vi "Toolbar Set Button Image (Picture).vi"(0 "Display State In":T2={"Buttons Displayed"=0, "Button States"=[], "Button Size"=0, "Button Style"=enum."Classic", "Active Button"=0, "Force Regen?"=FALSE, "Tip String Ref"=refnum}, 1 "Button Index":i32, 5 "State":T1, 7 "Picture":picture, 9 "Container State":T4, 11 "error in (no error)":errorcluster) -> (4 "Display State Out":T2={"Buttons Displayed"=0, "Button States"=[], "Button Size"=0, "Button Style"=enum."Classic", "Active Button"=0, "Force Regen?"=FALSE, "Tip String Ref"=refnum}, 15 "error out":errorcluster)   [LabVIEW 2012, in "Toolbar.xctl"]
doc: "Sets the image of specific button and state from a picture control."
uses:
  Toolbar.xctl
  <vilib>/_xctls/Container State.ctl
  Toolbar State.ctl
  Button_Class/Button.lvclass
  Button_Class/Type Defs/Button Style.ctl
  Button_Class/Type Defs/Button Status.ctl
  <vilib>/_xctls/XControlSupport.lvlib
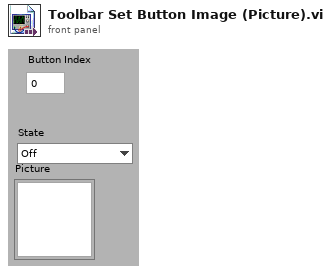
[diagram p1: front panel]
types:
  T1 = typedef "Button.lvclass/Button Status.ctl" = enum16{"Off", "Hover", "On", "Disabled"}
  T2 = typedef "Toolbar.xctl/Toolbar State.ctl" = cluster{"Buttons Displayed":i32, "Button States":refnum<class "Button.lvclass">[], "Button Size":i32, "Button Style":T3, "Active Button":i32, "Force Regen?":bool, "Tip String Ref":refnum<vi>}
  T3 = typedef "Button.lvclass/Button Style.ctl" = enum16{"System", "Modern", "Classic", "Rounded", "Silver", "Ni Theme", "Metallic"}
  T4 = typedef "XControlSupport.lvlib/Container State.ctl" = cluster{"Indicator?":bool, "Run Mode?":bool, " Refnum":refnum<vi>}
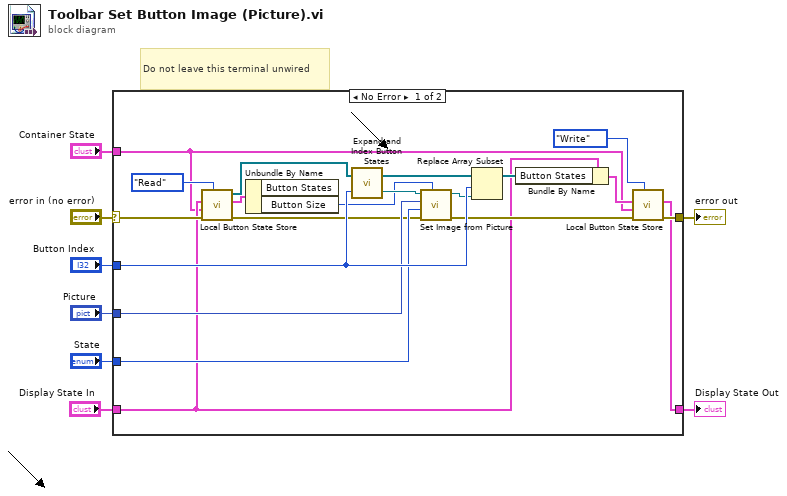
[diagram p0: block diagram]
diagram:
  # "Do not leave this terminal unwired"
  n1 = case shown="No Error" "error in (no error)" {
    selector: "error in (no error)" -> [w17 w29]
    tunnel: "Display State In" -> [w14 w30]
    tunnel: [w10 w30] -> w2
    tunnel: [w20 w29] -> w3
    tunnel: "Button Index" -> [w28 _]
    tunnel: "Picture" -> [w24 _]
    tunnel: "State" -> [w23 _]
    tunnel: "Container State" -> [w11 _]
    frame No Error {
      n2 = call "Local Button State Store.vi"("Operation"=enum16{"Read", "Write"}."Read", "error in (no error)"=w17, "Container State"=w11, "Display State In"=w14) -> ("error out"=w16:errorcluster, "Display State Out"=w13:T2, "Button States"=w9:refnum<class "Button.lvclass">[])  [unwired: 5 out]
      n3 = Unbundle By Name(w13) -> ("Button Size"=w22:i32)  [unwired: 1 out]
      n4 = call "Expand and Index Button States.vi"("Button Index"=w28, "Button States"=w9) -> ("Button.lvclass"=w26:refnum<class "Button.lvclass">, "Button States Out"=w27:refnum<class "Button.lvclass">[])
      n5 = call-dynamic "Set Image from Picture.vi"("Button Size"=w22, "error in (no error)"=w16, "State"=w23, "Picture"=w24, "Button in"=w26) -> ("error out"=w21:errorcluster, "Button out"=w25:refnum<class "Button.lvclass">)  [unwired: 5 out]
      n6 = Replace Array Subset(array=w27, new element=w25, index=w28) -> (w18:refnum<class "Button.lvclass">[])
      n7 = Bundle By Name(cluster=w14, "Button States"=w18) -> (w12:T2)
      n8 = call "Local Button State Store.vi"("Operation"=enum16{"Read", "Write"}."Write", "error in (no error)"=w21, "Container State"=w11, "Display State In"=w12) -> ("error out"=w20:errorcluster, "Display State Out"=w10:T2)  [unwired: 1 in, 5 out]
    }
    frame Error {
    }
  }
  "Display State Out" <- w2
  "error out" <- w3
